vi "AvoidWall.vi"(3 "SupressIn":dbl, 7 "Inhibit":bool, 8 "HowAmI? Clean":cluster{"T":dbl, "Battery":dbl, "Temp":dbl}, 9 "WhatAroundMe? Clean":cluster{"T":dbl, "Range":dbl, "Bearing":dbl}[](array[cluster]), 10 "WhereAmI? Clean":T1, 11 "Velocity":dbl) -> (0 "SupressOut":dbl, 2 "ActCommand":dbl[](array[numeric]))   [LabVIEW 2010]
doc: "This subVI behavior avoids walls parallel to teh direction of the robot. It does so by finding the centroid of the LIDAR data if the robot is within 20 pixels of the wall and placing a noraml distribution at that point.\n\nIt is designed to work with a 90 element behavior arbiter."
uses:
  <vilib>/Analysis/2dsp.llb/Integral Method.ctl
  <vilib>/Analysis/1siggen.llb/Ramp Pattern by Samples.vi
  <vilib>/Analysis/8numeric.llb/1D Numeric Integration.vi
  <vilib>/gmath/statdist.llb/Normal PDF.vi
  <vilib>/Analysis/NI_AALPro.lvlib
  <vilib>/gmath/NI_Gmath.lvlib
  <vilib>/Analysis/NI_AALBase.lvlib
panel:
  out "x+y":dbl
  out "Waveform Graph":dbl[][](graph)
  # "This contains a behavior that steers away from walls when they are too close"
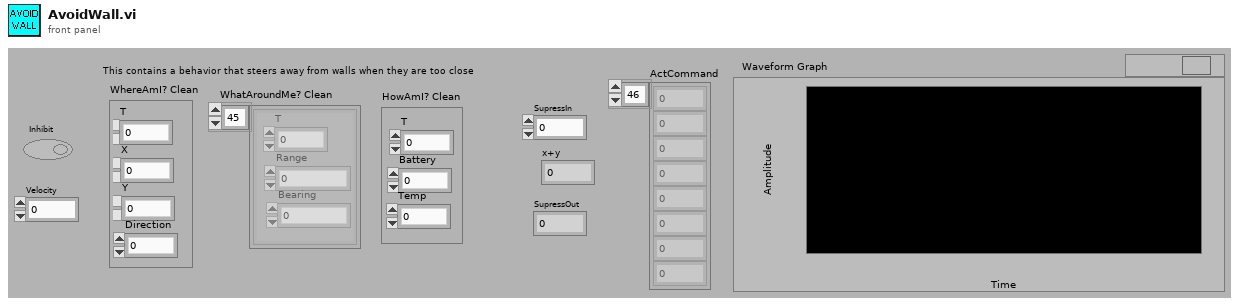
[diagram p1: front panel]
types:
  T1 = cluster{"T":dbl, "X":dbl, "Y":dbl, "Direction":dbl}
  T2 = typedef "NI_AALPro.lvlib/Integral Method.ctl" = i32
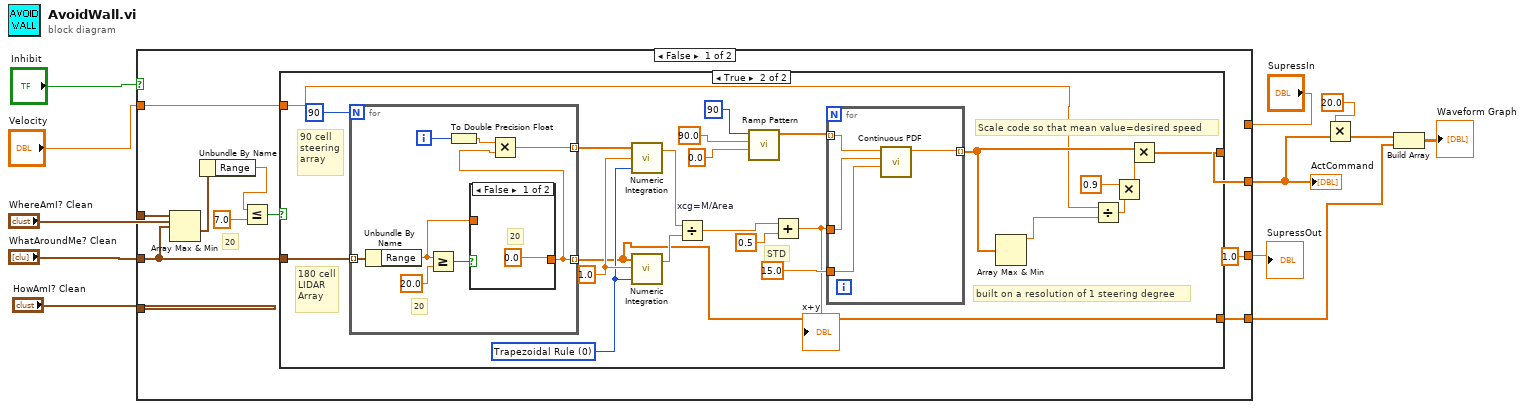
[diagram p0: block diagram]
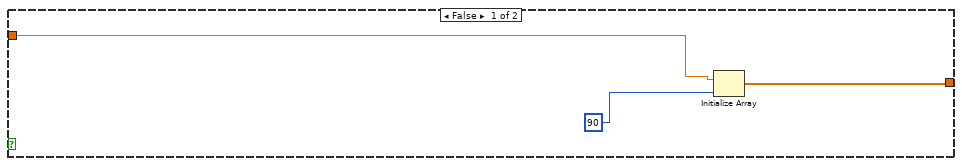
[diagram p2: hidden frame]
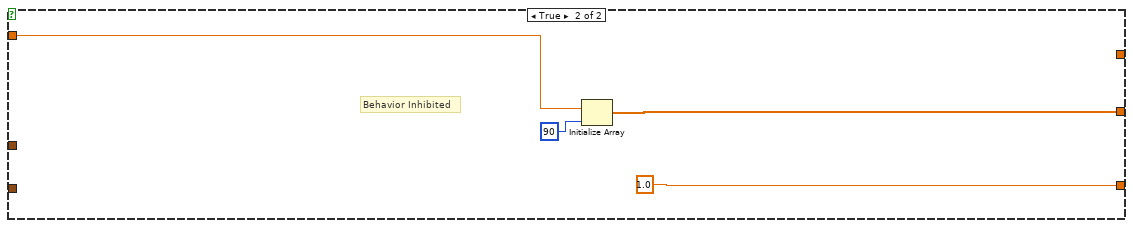
[diagram p4: hidden frame]
diagram:
  n1 = case shown="False" "Inhibit" {
    tunnel: "Velocity" -> [w19 w62]
    tunnel: "WhatAroundMe? Clean" -> [w17 _]
    tunnel: "WhereAmI? Clean" -> [_ _]
    tunnel: "HowAmI? Clean" -> [_ _]
    tunnel: "SupressIn" -> [_ _]
    tunnel: [w20 w63] -> w5
    tunnel: [1.0 ("SupressOut") 1.0 ("SupressOut")] -> w6
    tunnel: [w18 _] -> w3
    frame False {
      # "20"
      n2 = Array Max & Min(array=w17) -> (min value=w16:cluster{"T":dbl, "Range":dbl, "Bearing":dbl})  [unwired: 3 out]
      n3 = Unbundle By Name(w16) -> ("Range"=w14:dbl)
      n4 = Less Or Equal?(x=w14, y=7.0) -> (x <= y?=w15:bool)
      n5 = case shown="True" w15 {
        tunnel: w17 -> [_ w46]
        tunnel: [w23 w34] -> w20
        tunnel: w19 -> [w22 w32]
        tunnel: [_ w28] -> w18
        frame False {
          n6 = Initialize Array "Initialize Array"(w22, 90 ("dimension size")) -> (w23:dbl[])
        }
        frame True {
          w44 = 1.0 ("dt")
          w43 = T2 0 items=["Trapezoidal Rule", "Simpson's Rule", "Simpson's 3/8 Rule", "Bode Rule"] ("integration method")
          # "built on a resolution of 1 steering degree"
          # "Scale code so that mean value=desired speed"
          # "STD"
          # "180 cell\nLIDAR \nArray"
          # "90 cell\nsteering\narray"
          n7 = for {
            N: 90 -> [_]
            tunnel: w46 -> [w59] mode=indexing
            tunnel: [w54] -> w28 mode=indexing
            tunnel: [w52] -> w45 mode=indexing
            i -> [w55]
            # "20"
            n8 = Unbundle By Name(w59) -> ("Range"=w56:dbl)
            n9 = Greater Or Equal?(x=w56, y=20.0) -> (x >= y?=w57:bool)
            n10 = To Double Precision Float(number=w55) -> (double precision float=w53:dbl)
            n11 = case shown="False" w57 {
              tunnel: w56 -> [_ w61]
              tunnel: [0.0 ("Range") w61] -> w54
              frame False {
                # "20"
              }
              frame True {
              }
            }
            n12 = Multiply(x=w53, y=w54) -> (x*y=w52:dbl)
          }
          n13 = call-poly <vilib>:"Numeric Integration.vi"("integration method"=w43, "dt"=w44, "Input Array"=w45) -> ("result"=w33:dbl)  [unwired: 1 out]
          n14 = call-poly <vilib>:"Numeric Integration.vi"("integration method"=w43, "dt"=w44, "Input Array"=w28) -> ("result"=w42:dbl)  [unwired: 1 out]
          n15 = Divide "xcg=M/Area"(x=w33, y=w42) -> (x/y=w31:dbl)
          n16 = call-poly <vilib>:"Ramp Pattern.vi"("start"=0.0, "end"=90.0 ("end (Normal)"), "samples"=90) -> ("Ramp Pattern"=w27:dbl[])  [unwired: 7 in, 1 out]
          n17 = Add(x=w31, y=0.5) -> (x+y=w30:dbl)
          "x+y" <- w30
          n18 = for {
            tunnel: w27 -> [w51] mode=indexing
            tunnel: 15.0 ("std (Normal)") -> [w50]
            tunnel: [w49] -> w40 mode=indexing
            tunnel: w30 -> [w48]
            n19 = call-poly <vilib>:"Continuous PDF.vi"("std"=w50, "mean"=w48, "x"=w51) -> ("pdf(x)"=w49:dbl)  [unwired: 7 in, 1 out]
          }
          n20 = Array Max & Min(array=w40) -> (max value=w38:dbl)  [unwired: 3 out]
          n21 = Divide(x=w32, y=w38) -> (x/y=w39:dbl)
          n22 = Multiply(x=0.9, y=w39) -> (x*y=w26:dbl)
          n23 = Multiply(x=w40, y=w26) -> (x*y=w34:dbl[])
        }
      }
    }
    frame True {
      # "Behavior Inhibited"
      n24 = Initialize Array "Initialize Array"(w62, 90 ("dimension size")) -> (w63:dbl[])
    }
  }
  "ActCommand" <- w5
  "SupressOut" <- w6
  n25 = Multiply(x=20.0, y=w5) -> (x*y=w2:dbl[])
  n26 = Build Array(w2, w3) -> (→"Waveform Graph":dbl[][])
